vi "Set Control Effort.vi"(7 "Max Effort":i32=1000, 8 "error in (no error)":errorcluster, 9 "Motor2 Effort":i32, 10 "Motor1 Effort":i32, 11 "VISA resource name":refnum<visa-resource-name>) -> (0 "error out":errorcluster, 2 "Command":string, 3 "VISA resource name out":refnum<visa-resource-name>)   [LabVIEW 2012, in "Roboteq.lvlib"]
uses:
  Roboteq.lvlib
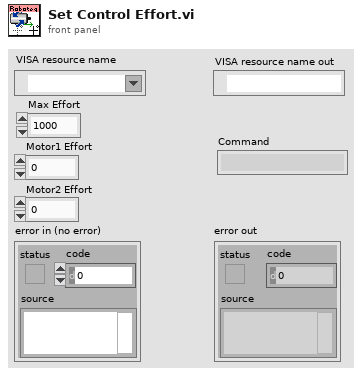
[diagram p1: front panel]
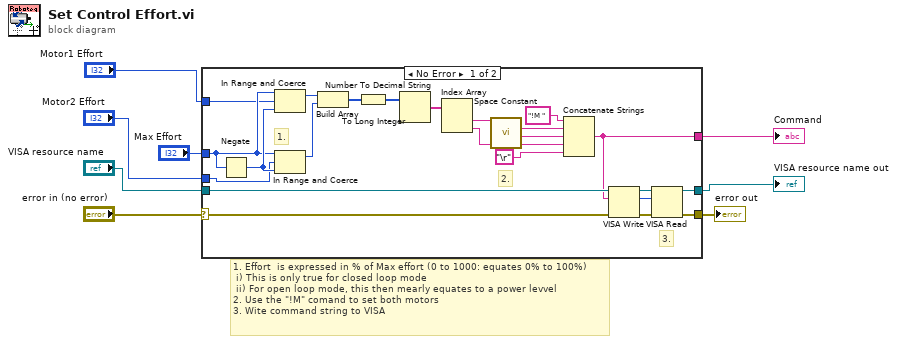
[diagram p0: block diagram]
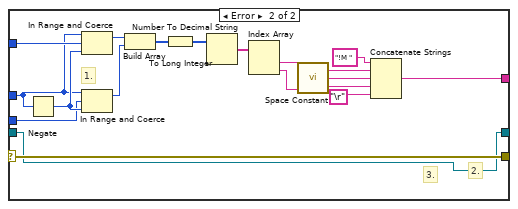
[diagram p2: hidden frame]
diagram:
  # "1. Effort  is expressed in % of Max effort (0 to 1000: equates 0% to 100%)\n i) This is only true for closed loop mode\n ii) For open loop mode, this then mearly equates to a power levvel \n2. Use the \"!M\" comand to set both motors\n3. Wite command string to VISA"
  n1 = case shown="No Error" "error in (no error)" {
    selector: "error in (no error)" -> [w21 w47]
    tunnel: "VISA resource name" -> [w20 w46]
    tunnel: [w9 w46] -> w7
    tunnel: [w10 w47] -> w6
    tunnel: "Motor1 Effort" -> [w15 w34]
    tunnel: "Motor2 Effort" -> [w14 w32]
    tunnel: [w19 w31] -> w2
    tunnel: "Max Effort" -> [w16 w33]
    frame No Error {
      # "3."
      # "2."
      # "1."
      n2 = Negate(x=w16) -> (-x=w30:i32)
      n3 = In Range and Coerce(upper limit=w16, x=w15, lower limit=w30) -> (coerced(x)=w29:i32)  [unwired: 1 out]
      n4 = In Range and Coerce(upper limit=w16, x=w14, lower limit=w30) -> (coerced(x)=w28:i32)  [unwired: 1 out]
      n5 = Build Array(w29, w28) -> (w18:i32[])
      n6 = To Long Integer(number=w18) -> (32bit integer=w17:i32[])
      n7 = Number To Decimal String(number=w17) -> (decimal integer string=w27:string[])  [unwired: 1 in]
      n8 = Index Array(array=w27) -> (element #1=w24:string, element #2=w23:string)  [unwired: 2 in]
      n9 = call <vilib>:"Space Constant.vi"() -> ("String"=w26:string)
      n10 = Concatenate Strings("!M " ("string"), w24, w26, w23, "\r") -> (w19:string)
      n11 = VISA Write(VISA resource name=w20, write buffer=w19, error in (no error)=w21) -> (VISA resource name out=w12:refnum<visa-resource-name>, return count=w13:u32, error out=w11:errorcluster)
      n12 = VISA Read(VISA resource name=w12, byte count=w13, error in (no error)=w11) -> (VISA resource name out=w9:refnum<visa-resource-name>, error out=w10:errorcluster)  [unwired: 2 out]
    }
    frame Error {
      # "3."
      # "2."
      # "1."
      n13 = Negate(x=w33) -> (-x=w45:i32)
      n14 = In Range and Coerce(upper limit=w33, x=w34, lower limit=w45) -> (coerced(x)=w44:i32)  [unwired: 1 out]
      n15 = In Range and Coerce(upper limit=w33, x=w32, lower limit=w45) -> (coerced(x)=w43:i32)  [unwired: 1 out]
      n16 = Build Array(w44, w43) -> (w36:i32[])
      n17 = To Long Integer(number=w36) -> (32bit integer=w35:i32[])
      n18 = Number To Decimal String(number=w35) -> (decimal integer string=w42:string[])  [unwired: 1 in]
      n19 = Index Array(array=w42) -> (element #1=w39:string, element #2=w38:string)  [unwired: 2 in]
      n20 = call <vilib>:"Space Constant.vi"() -> ("String"=w41:string)
      n21 = Concatenate Strings("!M " ("string"), w39, w41, w38, "\r") -> (w31:string)
    }
  }
  "VISA resource name out" <- w7
  "error out" <- w6
  "Command" <- w2
